vi "FPGA Main Simple Torque.vi"() -> ()   [LabVIEW 2018]
doc: "This VI reads all analogue data channels available at the fastest rate supported by the respective hardware and updates a memory address for when each measurement is available.\n\nAt a rate defined by the fastest module (NI 9237 - default of 12.5kHz) this memory is read, combined with the measurements from the 9237 module and written to the FIFO for communication to the RT machine.\n\nThe NI 9237 modeul therefore defines the nominal sampling rate of the system (with slower channels over-sampled).\n\nA time channel (in uSec) is provided with 0 referenced from the first acquisition of the NI 9237 module"
uses:
  <vilib>/LabVIEW Targets/FPGA/cRIO/shared/nicrio_ModuleControls/nicrio_cRIO-9237_DataRatesRing.ctl
  <vilib>/Platform/TimedLoop/XDataNode/timing_clust.ctl
  <vilib>/Platform/TimedLoop/XDataNode/nitl_modes.ctl
  <vilib>/Platform/TimedLoop/XDataNode/wakeup.ctl
  <vilib>/rvi/Emulation/niFpgaGetClockAttributes.vi
  <vilib>/rvi/Emulation/niFpgaSctlEmulationGetInTimedLoop.vi
  <vilib>/rvi/Emulation/niFpgaEmulationReportErrorSimple.vi
  <vilib>/rvi/Emulation/niFpgaProcessEmulError.vi
  <vilib>/rvi/eio/common/nirviEmuTemplatePropertySet_noerrors.vi
  <vilib>/rvi/eio/common/nirviEmuTemplateMethod_errors.vi
  <vilib>/rvi/interface/RandomDataEmulation/niFpgaRandomDataHandleErrors.vi
  <vilib>/rvi/Memory/Memory_Emulation/nirvimemoryFastEmulation.vi
  <vilib>/rvi/Memory/Memory_Emulation/nirvimemoryEmulation.vi
  <vilib>/rvi/Emulation/niFpgaEmulationIsFPGAContextNoSignature.vi
  <vilib>/rvi/DataTransferAndStorage/Container/Common/niFpgaContainerGetUniqueNameForEmu.vi
  <vilib>/rvi/errors/nirviReportUnexpectedCaseInternalError (U32).vi
  <vilib>/rvi/Emulation/niFpgaCriticalErrorInLSC.vi
  <vilib>/eio/EIOPropertyNode/EIOPropertyNode.xnode
  <vilib>/eio/EIONode/EIONode.xnode
  <vilib>/rvi/DataTransferAndStorage/Container/XNode/niFpgaContainer.xnode
  <vilib>/rvi/interface/RandomDataEmulation/nirviRandomDataFpgaReadWriteTemplate.vi
  <vilib>/platform/TimedLoop/XDataNode/XDataNode.xnode
  <vilib>/eio/EIOMethodNode/EIOMethodNode.xnode
  <vilib>/Platform/TimedLoop/XDataNode/XDNodeRunTimeDep.lvlib
  <vilib>/rvi/eio/common/nirviEmuTemplatePropertyGet_errors.vi
  <vilib>/rvi/eio/common/nirviEmuTemplatePropertyGet_noerrors.vi
  <vilib>/rvi/eio/common/nirviEmuTemplatePropertySet_errors.vi
panel:
  in  "filterTorque":bool
  in  "Data Rate":T1=1 items=["50.000 kS/s (NI 9237)"=1, "25.000 kS/s (NI 9237)"=2, "16.667 kS/s (NI 9237)"=3, "12.500 kS/s (NI 9237)"=4, "10.000 kS/s (NI 9237)"=5, "8.333 kS/s (NI 9237)"=6, "7.143 kS/s (NI 9237)"=7, "6.250 kS/s (NI 9237)"=8, "5.556 kS/s (NI 9237)"=9, "5.000 kS/s (NI 9237)"=10, "4.545 kS/s (NI 9237)"=11, "4.167 kS/s (NI 9237)"=12, "3.846 kS/s (NI 9237)"=13, "3.571 kS/s (NI 9237)"=14, "3.333 kS/s (NI 9237)"=15, "3.125 kS/s (NI 9237)"=16, "2.941 kS/s (NI 9237)"=17, "2.778 kS/s (NI 9237)"=18, "2.632 kS/s (NI 9237)"=19, "2.500 kS/s (NI 9237)"=20, "2.381 kS/s (NI 9237)"=21, "2.273 kS/s (NI 9237)"=22, "2.174 kS/s (NI 9237)"=23, "2.083 kS/s (NI 9237)"=24, "2.000 kS/s (NI 9237)"=25, "1.923 kS/s (NI 9237)"=26, "1.852 kS/s (NI 9237)"=27, "1.786 kS/s (NI 9237)"=28, "1.724 kS/s (NI 9237)"=29, "1.667 kS/s (NI 9237)"=30, "1.613 kS/s (NI 9237)"=31]
  in  "encoders offset":u32 caption="encoder offset @ 1Hz (ticks)"
  out "Total channel count":u32=61
  out "timestamp":u32
  out "FIFO full counter":i32
  in  "Safe Voltage":fxp<+/-,20,5>[](array[numeric])=[0.0, 0.0, 0.0, 0.0]
  in  "Safe Digital":bool[](array[boolean])=[FALSE, FALSE, FALSE, FALSE, FALSE, FALSE, FALSE, FALSE]
  in  "Voltage Out":fxp<+/-,20,5>[](array[numeric])=[0.0, 0.0, 0.0, 0.0]
  in  "Update Outputs":bool
  in  "Mod 8":bool[](array[boolean])=[FALSE, FALSE, FALSE, FALSE, FALSE, FALSE, FALSE, FALSE]
  out "E Stop":bool
  in  "Stop acquire":bool
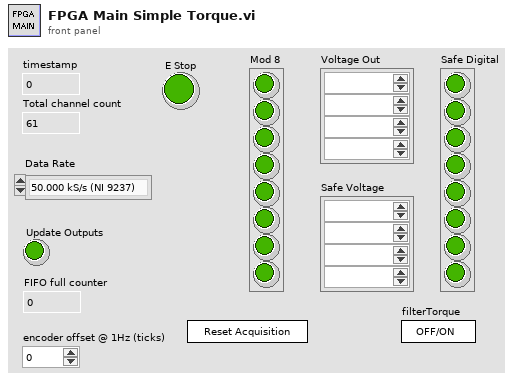
[diagram p1: front panel]
types:
  T1 = typedef "nicrio_cRIO-9237_DataRatesRing.ctl" = u8
  T2 = typedef "XDNodeRunTimeDep.lvlib/timing_clust.ctl" = cluster{"Expected End [f-1]":u64, "Actual End [f-1]":u64, "Finished Late? [f-1]":bool, "Expected End [i-1]":u64, "Actual End [i-1]":u64, "Finished Late? [i-1]":bool, "Expected Start [i]":u64, "Actual Start [i]":u64, "Expected Start [f]":u64, "Actual Start [f]":u64, "Source Name":string, "Structure Name":string, "Period":i64, "Deadline":i64, "Offset":i64, "Start":i64, "Priority":i32, "Timeout":i32, "Mode":T3, "Wakeup Reason":T4, "Error":errorcluster, "Source Type":string, "Secondary Source Type":string, "Global End Time":u64, "Global Start Time":u64, "Frame Duration":u64, "Iteration Duration":u64, "Assigned CPU":i32, "I/O Scan Engine Mode":u32}
  T3 = typedef "XDNodeRunTimeDep.lvlib/nitl_modes.ctl" = enum32{"No Change", "Process missed periods, maintain original phase", "Discard missed periods, maintain original phase", "Process missed periods, ignore original phase", "Discard missed periods, ignore original phase"}
  T4 = typedef "XDNodeRunTimeDep.lvlib/wakeup.ctl" = enum32{"Normal", "Aborted", "Asynchronous wakeup", "Timing source error", "Timed loop error", "Timeout"}
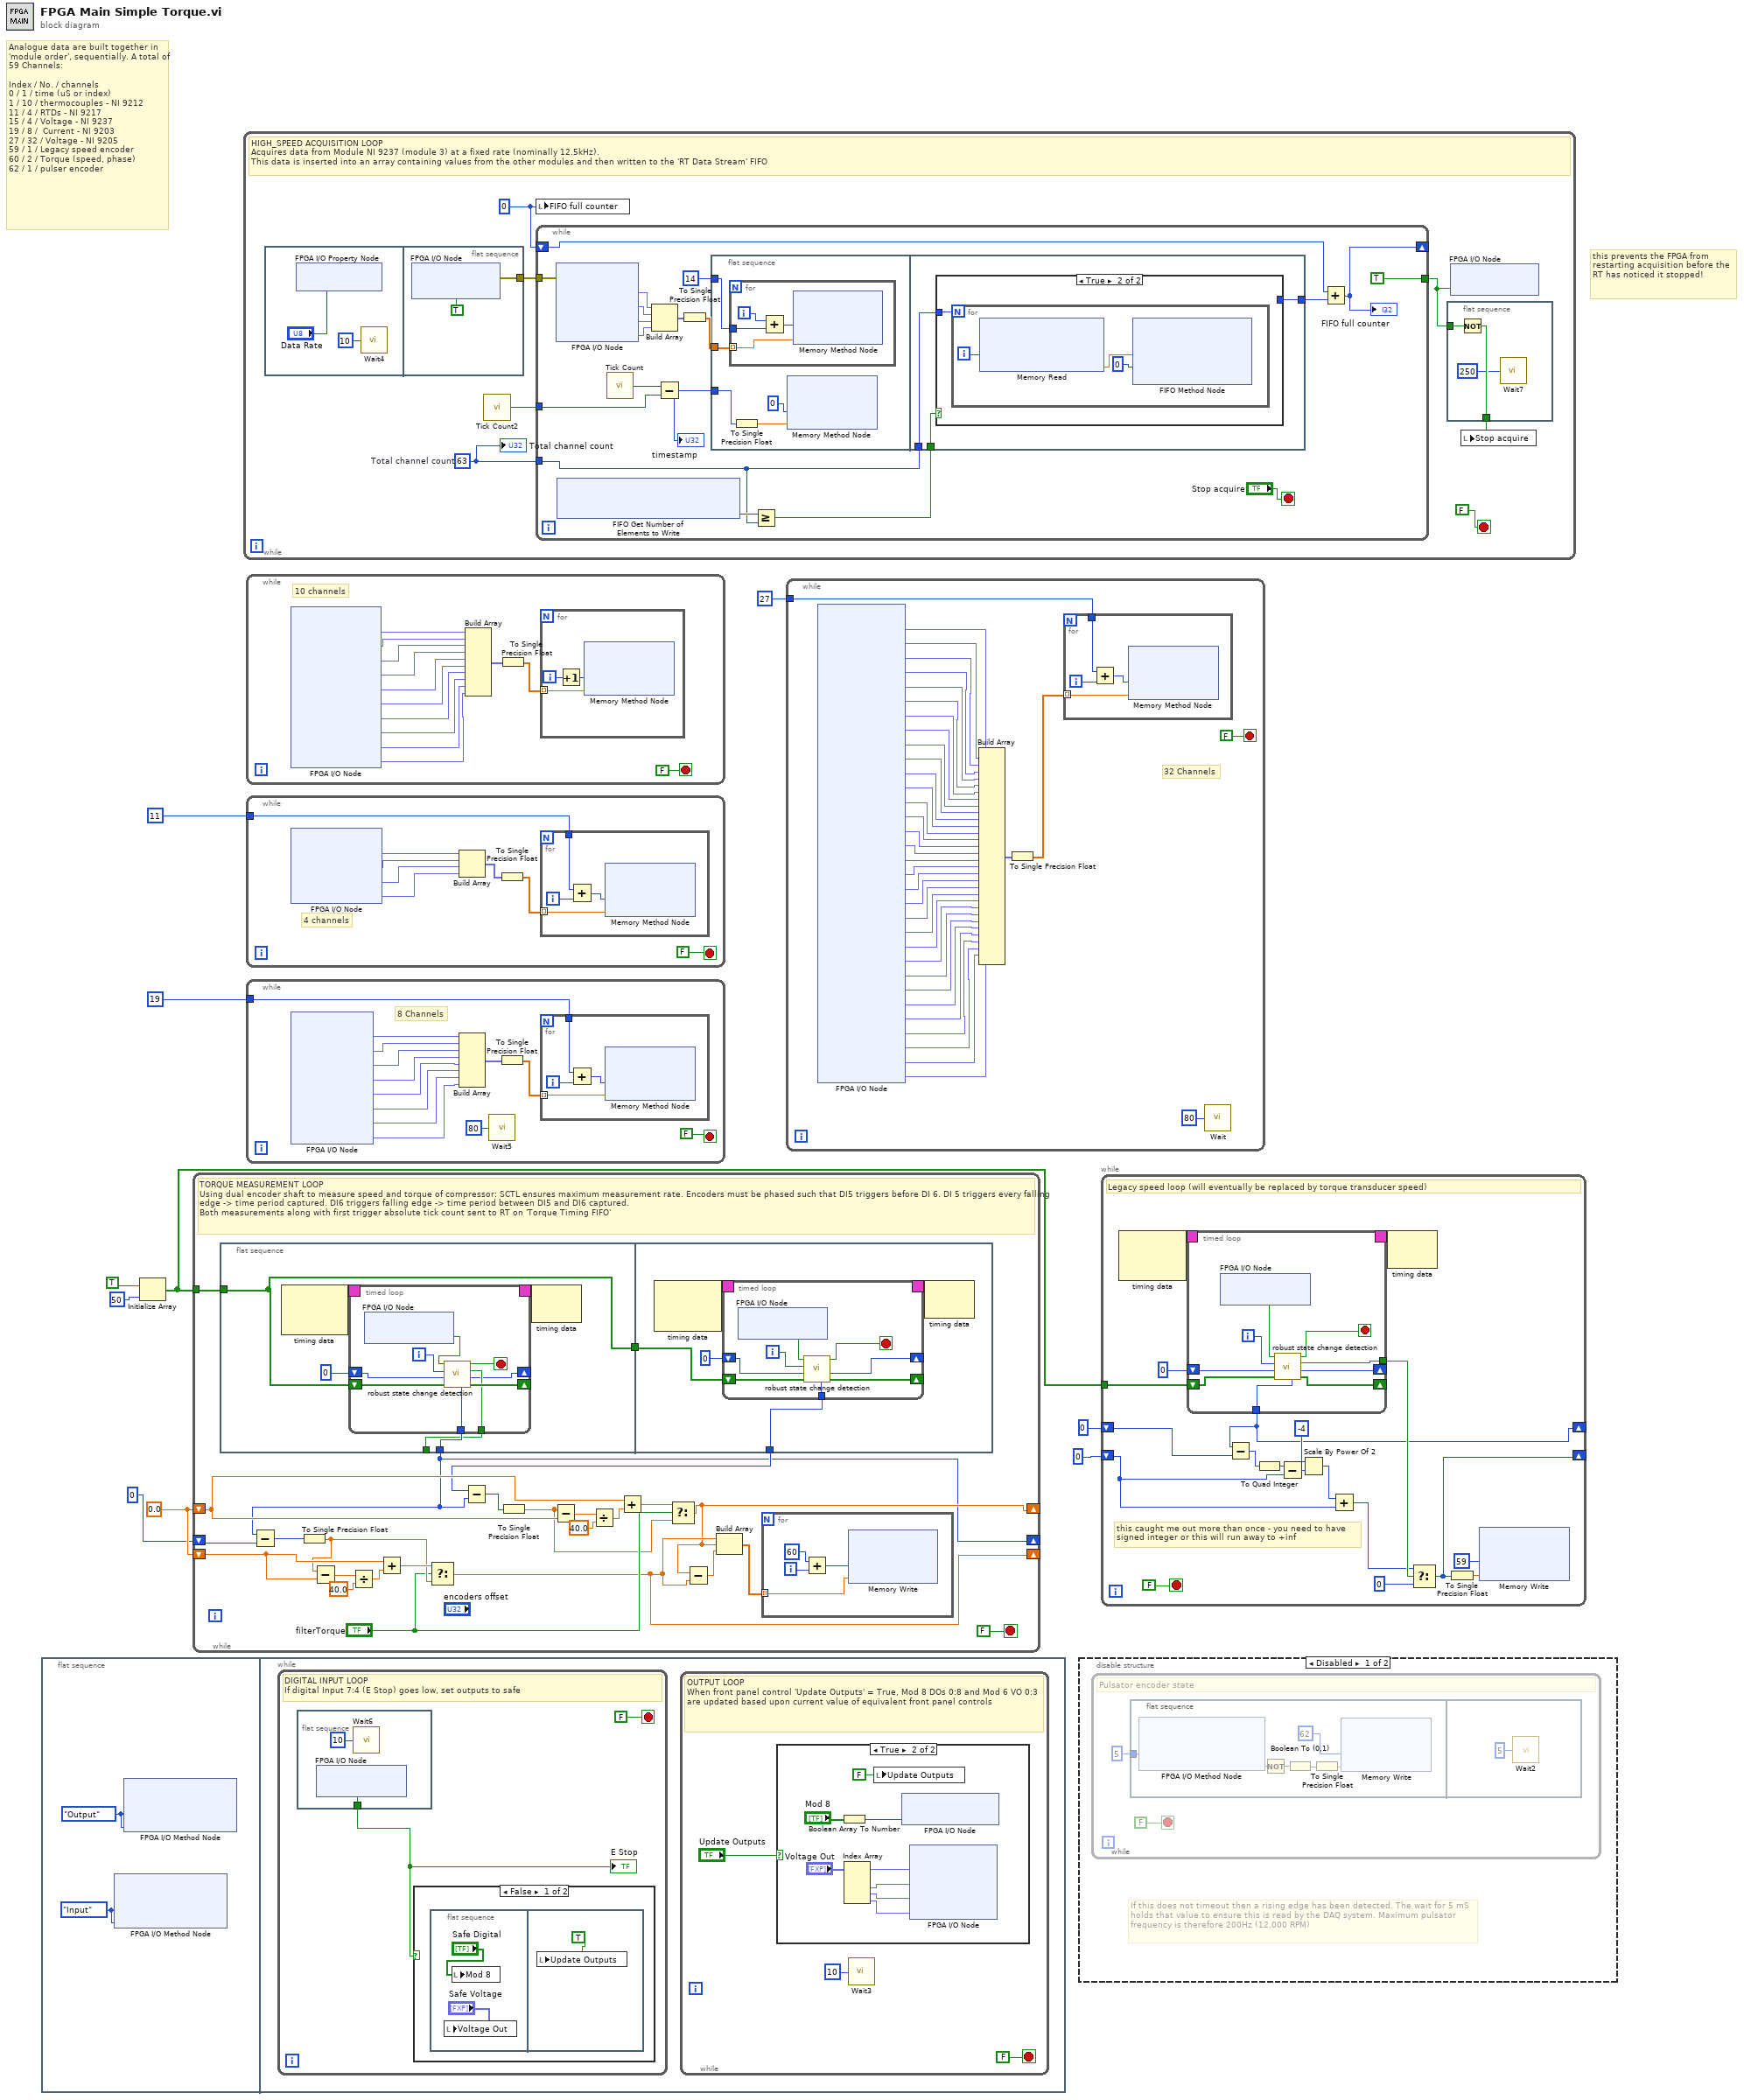
[diagram p0: block diagram]
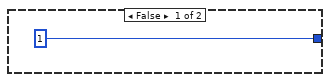
[diagram p5: hidden frame]
diagram:
  w2 = sgl 0.0
  # "this prevents the FPGA from restarting acquisition before the RT has noticed it stopped!"
  # "Analogue data are built together in 'module order', sequentially. A total of 59 Channels:\n\nIndex / No. / channels\n0 / 1 / time (uS or index)\n1 / 10 / thermocouples - NI 9212\n11 / 4 / RTDs - NI 9217\n15 / 4 / Voltage - NI 9237\n19 / 8 /  Current - NI 9203\n27 / 32 / Voltage - NI 9205\n59 / 1 / Legacy speed encoder\n60 / 2 / Torque (speed, phase)\n62 / 1 / pulser encoder"
  n1 = flat-sequence {
    frame #0 {
      w11 = enum8{"No Change", "Input", "Output"}."Output" ("DIO 7:4")
      w12 = enum8{"No Change", "Input", "Output"}."Input" ("DIO 7:4")
      n2 = xnode "FPGA I/O Method Node"("DIO 7:4"=w12, "DIO 3:0"=w12) -> ()  [unwired: 1 in, 1 out]
      n3 = xnode "FPGA I/O Method Node"("DIO 7:4"=w11, "DIO 3:0"=w11) -> ()  [unwired: 1 in, 1 out]
    }
    frame #1 {
      n4 = while {
        stop <- FALSE stop-if-true
        # "DIGITAL INPUT LOOP\nIf digital Input 7:4 (E Stop) goes low, set outputs to safe"
        n5 = flat-sequence {
          tunnel: [w27] -> w24
          frame #0 {
            n6 = xnode "FPGA I/O Node"() -> ("Mod7/DIO4"=w27:bool)  [unwired: 1 in, 1 out]
            n7 = call "Wait6"("Count(uSec)"=u8 10) -> ()  [unwired: 1 out]
          }
        }
        n8 = case shown="False" w24 {
          frame False {
            n9 = flat-sequence {
              frame #0 {
                n10 = local write "Voltage Out"("Safe Voltage") -> ()
                n11 = local write "Mod 8"("Safe Digital") -> ()
              }
              frame #1 {
                n12 = local write "Update Outputs"(TRUE ("Update Outputs")) -> ()
              }
            }
          }
          frame True {
          }
        }
        "E Stop" <- w24
      }
      n13 = while {
        stop <- FALSE stop-if-true
        # "OUTPUT LOOP\nWhen front panel control 'Update Outputs' = True, Mod 8 DOs 0:8 and Mod 6 VO 0:3 are updated based upon current value of equivalent front panel controls"
        n14 = case shown="True" "Update Outputs" {
          frame False {
          }
          frame True {
            n15 = Boolean Array To Number(Boolean array="Mod 8") -> (number=w22:u8)
            n16 = Index Array(array="Voltage Out") -> (element #1=w20:fxp<+/-,20,5>, element #2=w19:fxp<+/-,20,5>, element #3=w18:fxp<+/-,20,5>, element #4=w17:fxp<+/-,20,5>)  [unwired: 4 in]
            n17 = local write "Update Outputs"(FALSE ("Update Outputs")) -> ()
            n18 = xnode "FPGA I/O Node"("Mod8/DIO7:0"=w22) -> ()  [unwired: 1 in, 1 out]
            n19 = xnode "FPGA I/O Node"("Mod6/AO0"=w20, "Mod6/AO1"=w19, "Mod6/AO2"=w18, "Mod6/AO3"=w17) -> ()  [unwired: 4 in, 4 out]
          }
        }
        n20 = call "Wait3"("Count(uSec)"=u16 10 ("Count(Ticks)")) -> ()  [unwired: 1 out]
      }
    }
  }
  n21 = Initialize Array(TRUE, 50 ("edge buffer size")) -> (w4:bool[])
  n22 = while {
    shift-right: [w33] -> _
    shift-left: w2 -> [w43]
    shift-right: [w32] -> _
    shift-left: w2 -> [w53]
    tunnel: w4 -> [w52]
    shift-right: [w31] -> _
    shift-left: u32 0 ("tick") -> [w37]
    stop <- FALSE stop-if-true
    # "TORQUE MEASUREMENT LOOP\nUsing dual encoder shaft to measure speed and torque of compressor: SCTL ensures maximum measurement rate. Encoders must be phased such that DI5 triggers before DI 6. DI 5 triggers every falling edge -> time period captured. DI6 triggers falling edge -> time period between DI5 and DI6 captured.\nBoth measurements along with first trigger absolute tick count sent to RT on 'Torque Timing FIFO'"
    n23 = flat-sequence {
      tunnel: [w63] -> w31
      tunnel: [w62] -> _
      tunnel: w52 -> [w60]
      tunnel: [w60] -> w51
      tunnel: [w83] -> w34
      tunnel: w51 -> [w82]
      frame #0 {
        n24 = node-c288() -> (w65:T2)  [unwired: 2 in]
        n25 = timed-loop {
          timing: w65 -> [_]
          timing-out: [_] -> w64
          tunnel: [w69] -> w63
          tunnel: [w68] -> w62
          shift-right: [w72] -> _
          shift-left: w60 -> [w73]
          shift-right: [w66] -> _
          shift-left: i16 0 ("step") -> [w70]
          i -> [w71]
          stop <- w67 stop-if-true
          n26 = xnode "FPGA I/O Node"() -> ("Mod7/DIO0"=w74:bool)  [unwired: 1 in, 1 out]
          n27 = call "robust state change detection.vi"("history"=w73, "step"=w70, "tick"=w71, "New state"=w74) -> ("history out"=w72:bool[], "step out"=w66:i16, "edge detected"=w68:bool, "Stop?"=w67:bool, "tick"=w69:u32)  [unwired: 3 in]
        }
        n28 = node-c288(w64) -> ()  [unwired: 1 out]
      }
      frame #1 {
        n29 = node-c288() -> (w81:T2)  [unwired: 2 in]
        n30 = timed-loop {
          timing: w81 -> [_]
          timing-out: [_] -> w80
          shift-right: [w89] -> _
          shift-left: w82 -> [w90]
          tunnel: [w87] -> w83
          shift-right: [w84] -> _
          shift-left: i16 0 ("step") -> [w85]
          i -> [w86]
          stop <- w88 stop-if-true
          n31 = xnode "FPGA I/O Node"() -> ("Mod7/DIO1"=w91:bool)  [unwired: 1 in, 1 out]
          n32 = call "robust state change detection.vi"("history"=w90, "step"=w85, "tick"=w86, "New state"=w91) -> ("history out"=w89:bool[], "step out"=w84:i16, "Stop?"=w88:bool, "tick"=w87:u32)  [unwired: 3 in, 1 out]
        }
        n33 = node-c288(w80) -> ()  [unwired: 1 out]
      }
    }
    n34 = Subtract(x=w31, y=w37) -> (x-y=w36:u32)
    n35 = To Single Precision Float(number=w36) -> (single precision float=w41:sgl)
    n36 = Subtract(x=w41, y=w43) -> (x-y=w44:sgl)
    n37 = Divide(x=w44, y=sgl 40.0) -> (x/y=w45:sgl)
    n38 = Add(x=w43, y=w45) -> (x+y=w46:sgl)
    n39 = Select(t=w46, s="filterTorque", f=w41) -> (s? t:f=w33:sgl)
    n40 = Subtract(x=w34, y=w31) -> (x-y=w35:u32)
    n41 = To Single Precision Float(number=w35) -> (single precision float=w39:sgl)
    n42 = Subtract(x=w39, y=w53) -> (x-y=w50:sgl)
    n43 = Divide(x=w50, y=sgl 40.0) -> (x/y=w48:sgl)
    n44 = Add(x=w53, y=w48) -> (x+y=w47:sgl)
    n45 = Select(t=w47, s="filterTorque", f=w39) -> (s? t:f=w32:sgl)
    n46 = Subtract(x=w32, y=w33) -> (x-y=w38:sgl)
    n47 = Build Array(w33, w32, w38) -> (w54:sgl[])
    n48 = for {
      tunnel: w54 -> [w56] mode=indexing
      i -> [w57]
      n49 = Add(x=u32 60 ("Address"), y=w57) -> (x+y=w58:u32)
      n50 = xnode ("Memory Write")("Address"=w58, "Data"=w56) -> ()  [unwired: 1 in, 1 out]
    }
  }
  n51 = while {
    stop <- FALSE stop-if-true
    w97 = 0 ("FIFO full counter")
    w100 = u32 63  # Total channel count
    # "HIGH_SPEED ACQUISITION LOOP\nAcquires data from Module NI 9237 (module 3) at a fixed rate (nominally 12.5kHz).\nThis data is inserted into an array containing values from the other modules and then written to the 'RT Data Stream' FIFO"
    n52 = flat-sequence {
      tunnel: [w109] -> w101
      frame #0 {
        n53 = xnode "FPGA I/O Property Node"("Data Rate"="Data Rate") -> ()  [unwired: 1 in, 1 out]
        n54 = call "Wait4"("Count(mSec)"=u16 10) -> ()  [unwired: 1 out]
      }
      frame #1 {
        n55 = xnode "FPGA I/O Node"("Mod3/Start"=TRUE) -> ("error out"=w109:errorcluster)  [unwired: 2 in, 1 out]
      }
    }
    n56 = call "Tick Count2"() -> ("Tick Count(uSec)"=w102:u32)
    n57 = local write "FIFO full counter"(w97) -> ()
    n58 = while {
      tunnel: [TRUE ("I/O Item")] -> w99
      tunnel: w101 -> [w127]
      tunnel: w100 -> [w112]
      shift-right: [w120] -> _
      shift-left: w97 -> [w118]
      tunnel: w102 -> [w121]
      stop <- "Stop acquire" stop-if-true
      n59 = xnode "FPGA I/O Node"("error in"=w127) -> ("Mod3/AI0"=w126:fxp<+/-,24,-4>, "Mod3/AI1"=w125:fxp<+/-,24,-4>, "Mod3/AI2"=w124:fxp<+/-,24,-4>, "Mod3/AI3"=w123:fxp<+/-,24,-4>)  [unwired: 4 in, 5 out]
      n60 = xnode ("FIFO Get Number of Elements to Write")() -> ("Number of Elements to Write"=w114:u32)  [unwired: 1 in, 1 out]
      n61 = call "Tick Count"() -> ("Tick Count(uSec)"=w117:u32)
      n62 = Build Array(w126, w125, w124, w123) -> (w122:fxp<+/-,24,-4>[])
      n63 = Subtract(x=w117, y=w121) -> (x-y=w110:u32)
      "timestamp" <- w110
      n64 = To Single Precision Float(number=w122) -> (single precision float=w116:sgl[])
      n65 = flat-sequence {
        tunnel: w116 -> [w133]
        tunnel: 14 ("index") -> [w132]
        tunnel: w110 -> [w130]
        tunnel: w112 -> [w140]
        tunnel: [w139] -> w111
        tunnel: w113 -> [w138]
        frame #0 {
          n66 = for {
            tunnel: w133 -> [w137] mode=indexing
            tunnel: w132 -> [w136]
            i -> [w134]
            n67 = Add(x=w134, y=w136) -> (x+y=w135:i32)
            n68 = xnode ("Memory Method Node")("Address"=w135, "Data"=w137) -> ()  [unwired: 1 in, 1 out]
          }
          n69 = To Single Precision Float(number=w130) -> (single precision float=w131:sgl)
          n70 = xnode ("Memory Method Node")("Address"=u32 0, "Data"=w131) -> ()  [unwired: 1 in, 1 out]
        }
        frame #1 {
          n71 = case shown="True" w138 {
            tunnel: [1 _] -> w139
            tunnel: w140 -> [_ w142]
            frame False {
            }
            frame True {
              n72 = for {
                N: w142 -> [_]
                i -> [w143]
                n73 = xnode ("Memory Read")("Address"=w143) -> ("Data"=w144:sgl)  [unwired: 1 in, 1 out]
                n74 = xnode ("FIFO Method Node")("Element"=w144, "Timeout"=0) -> ()  [unwired: 1 in, 2 out]
              }
            }
          }
        }
      }
      n75 = Greater Or Equal?(x=w114, y=w112) -> (x >= y?=w113:bool)
      n76 = Add(x=w118, y=w111) -> (x+y=w120:i32)
      "FIFO full counter" <- w120
    }
    n77 = flat-sequence {
      tunnel: w99 -> [w105]
      tunnel: [w104] -> w96
      frame #0 {
        n78 = Not(x=w105) -> (.not. x?=w104:bool)
        n79 = call "Wait7"("Count(mSec)"=u8 250) -> ()  [unwired: 1 out]
      }
    }
    n80 = xnode "FPGA I/O Node"("Mod3/Stop"=w99) -> ()  [unwired: 1 in, 1 out]
    n81 = local write "Stop acquire"(w96) -> ()
    "Total channel count" <- w100
  }
  n82 = while {
    stop <- FALSE stop-if-true
    # "10 channels"
    n83 = xnode "FPGA I/O Node"() -> ("Mod1/TC0"=w158:fxp<+/-,24,-2>, "Mod1/TC1"=w157:fxp<+/-,24,-2>, "Mod1/TC2"=w156:fxp<+/-,24,-2>, "Mod1/TC3"=w155:fxp<+/-,24,-2>, "Mod1/TC4"=w154:fxp<+/-,24,-2>, "Mod1/TC5"=w153:fxp<+/-,24,-2>, "Mod1/TC6"=w152:fxp<+/-,24,-2>, "Mod1/TC7"=w151:fxp<+/-,24,-2>, "Mod1/CJC0"=w148:fxp<+/-,24,-2>, "Mod1/CJC1"=w147:fxp<+/-,24,-2>)  [unwired: 10 in, 10 out]
    n84 = Build Array(w158, w157, w156, w155, w154, w153, w152, w151, w148, w147) -> (w150:fxp<+/-,24,-2>[])
    n85 = To Single Precision Float(number=w150) -> (single precision float=w149:sgl[])
    n86 = for {
      tunnel: w149 -> [w161] mode=indexing
      i -> [w160]
      n87 = Increment(x=w160) -> (x+1=w159:i32)
      n88 = xnode ("Memory Method Node")("Address"=w159, "Data"=w161) -> ()  [unwired: 1 in, 1 out]
    }
  }
  n89 = while {
    tunnel: 11 ("Numeric") -> [w163]
    stop <- FALSE stop-if-true
    # "4 channels"
    n90 = xnode "FPGA I/O Node"() -> ("Mod2/RTD0"=w169:fxp<+/-,24,10>, "Mod2/RTD1"=w168:fxp<+/-,24,10>, "Mod2/RTD2"=w167:fxp<+/-,24,10>, "Mod2/RTD3"=w164:fxp<+/-,24,10>)  [unwired: 4 in, 4 out]
    n91 = Build Array(w169, w168, w167, w164) -> (w166:fxp<+/-,24,10>[])
    n92 = To Single Precision Float(number=w166) -> (single precision float=w165:sgl[])
    n93 = for {
      tunnel: w165 -> [w173] mode=indexing
      tunnel: w163 -> [w170]
      i -> [w172]
      n94 = Add(x=w170, y=w172) -> (x+y=w171:i32)
      n95 = xnode ("Memory Method Node")("Address"=w171, "Data"=w173) -> ()  [unwired: 1 in, 1 out]
    }
  }
  n96 = while {
    tunnel: 19 ("Numeric") -> [w180]
    stop <- FALSE stop-if-true
    # "8 Channels"
    n97 = xnode "FPGA I/O Node"() -> ("Mod4/AI0"=w186:fxp<+/-,21,-4>, "Mod4/AI1"=w185:fxp<+/-,21,-4>, "Mod4/AI2"=w184:fxp<+/-,21,-4>, "Mod4/AI3"=w181:fxp<+/-,21,-4>, "Mod4/AI4"=w179:fxp<+/-,21,-4>, "Mod4/AI5"=w178:fxp<+/-,21,-4>, "Mod4/AI6"=w177:fxp<+/-,21,-4>, "Mod4/AI7"=w176:fxp<+/-,21,-4>)  [unwired: 8 in, 8 out]
    n98 = Build Array(w186, w185, w184, w181, w179, w178, w177, w176) -> (w183:fxp<+/-,21,-4>[])
    n99 = call "Wait5"("Count(uSec)"=u8 80) -> ()  [unwired: 1 out]
    n100 = To Single Precision Float(number=w183) -> (single precision float=w182:sgl[])
    n101 = for {
      tunnel: w182 -> [w190] mode=indexing
      tunnel: w180 -> [w187]
      i -> [w189]
      n102 = Add(x=w187, y=w189) -> (x+y=w188:i32)
      n103 = xnode ("Memory Method Node")("Address"=w188, "Data"=w190) -> ()  [unwired: 1 in, 1 out]
    }
  }
  n104 = while {
    tunnel: 27 ("Numeric") -> [w226]
    stop <- FALSE stop-if-true
    # "32 Channels"
    n105 = xnode "FPGA I/O Node"() -> ("Mod5/AI0"=w194:fxp<+/-,26,5>, "Mod5/AI1"=w195:fxp<+/-,26,5>, "Mod5/AI2"=w196:fxp<+/-,26,5>, "Mod5/AI3"=w197:fxp<+/-,26,5>, "Mod5/AI4"=w198:fxp<+/-,26,5>, "Mod5/AI5"=w199:fxp<+/-,26,5>, "Mod5/AI6"=w200:fxp<+/-,26,5>, "Mod5/AI7"=w201:fxp<+/-,26,5>, "Mod5/AI8"=w225:fxp<+/-,26,5>, "Mod5/AI9"=w224:fxp<+/-,26,5>, "Mod5/AI10"=w223:fxp<+/-,26,5>, "Mod5/AI11"=w222:fxp<+/-,26,5>, "Mod5/AI12"=w221:fxp<+/-,26,5>, "Mod5/AI13"=w220:fxp<+/-,26,5>, "Mod5/AI14"=w219:fxp<+/-,26,5>, "Mod5/AI15"=w218:fxp<+/-,26,5>, "Mod5/AI16"=w217:fxp<+/-,26,5>, "Mod5/AI17"=w216:fxp<+/-,26,5>, "Mod5/AI18"=w215:fxp<+/-,26,5>, "Mod5/AI19"=w214:fxp<+/-,26,5>, "Mod5/AI20"=w213:fxp<+/-,26,5>, "Mod5/AI21"=w212:fxp<+/-,26,5>, "Mod5/AI22"=w211:fxp<+/-,26,5>, "Mod5/AI23"=w210:fxp<+/-,26,5>, "Mod5/AI24"=w209:fxp<+/-,26,5>, "Mod5/AI25"=w208:fxp<+/-,26,5>, "Mod5/AI26"=w207:fxp<+/-,26,5>, "Mod5/AI27"=w206:fxp<+/-,26,5>, "Mod5/AI28"=w205:fxp<+/-,26,5>, "Mod5/AI29"=w204:fxp<+/-,26,5>, "Mod5/AI30"=w203:fxp<+/-,26,5>, "Mod5/AI31"=w202:fxp<+/-,26,5>)  [unwired: 32 in, 32 out]
    n106 = Build Array(w194, w195, w196, w197, w198, w199, w200, w201, w225, w224, w223, w222, w221, w220, w219, w218, w217, w216, w215, w214, w213, w212, w211, w210, w209, w208, w207, w206, w205, w204, w203, w202) -> (w227:fxp<+/-,26,5>[])
    n107 = To Single Precision Float(number=w227) -> (single precision float=w193:sgl[])
    n108 = for {
      tunnel: w193 -> [w231] mode=indexing
      tunnel: w226 -> [w228]
      i -> [w230]
      n109 = Add(x=w228, y=w230) -> (x+y=w229:i32)
      n110 = xnode ("Memory Method Node")("Address"=w229, "Data"=w231) -> ()  [unwired: 1 in, 1 out]
    }
    n111 = call "Wait"("Count(uSec)"=u8 80) -> ()  [unwired: 1 out]
  }
  n112 = disable-structure shown="Disabled" {
    frame Disabled {
      # "If this does not timeout then a rising edge has been detected. The wait for 5 mS holds that value to ensure this is read by the DAQ system. Maximum pulsator frequency is therefore 200Hz (12,000 RPM)"
      n113 = while {
        stop <- FALSE stop-if-true
        # "Pulsator encoder state"
        n114 = flat-sequence {
          tunnel: 5 ("Timeout") -> [w236]
          frame #0 {
            n115 = xnode "FPGA I/O Method Node"("Timeout"=w236) -> ("Timed Out"=w235:bool)  [unwired: 1 in, 1 out]
            n116 = Not(x=w235) -> (.not. x?=w234:bool)
            n117 = Boolean To (0,1)(Boolean=w234) -> (0, 1=w239:i16)
            n118 = To Single Precision Float(number=w239) -> (single precision float=w238:sgl)
            n119 = xnode ("Memory Write")("Address"=u32 62, "Data"=w238) -> ()  [unwired: 1 in, 1 out]
          }
          frame #1 {
            n120 = call "Wait2"("Count(mSec)"=u16 5 ("Count(uSec)")) -> ()  [unwired: 1 out]
          }
        }
      }
    }
    frame Enabled {
    }
  }
  n121 = while {
    shift-right: [w246] -> _
    shift-left: i64 0 -> [w253]
    tunnel: w4 -> [w247]
    shift-right: [w242] -> _
    shift-left: u32 0 ("tick") -> [w241]
    stop <- FALSE stop-if-true
    # "this caught me out more than once - you need to have signed integer or this will run away to +inf"
    # "Legacy speed loop (will eventually be replaced by torque transducer speed)"
    n122 = node-c288() -> (w259:T2)  [unwired: 2 in]
    n123 = timed-loop {
      timing: w259 -> [_]
      timing-out: [_] -> w258
      shift-right: [w265] -> _
      shift-left: i16 0 ("step") -> [w266]
      tunnel: [w263] -> w248
      tunnel: [w262] -> w242
      shift-right: [w260] -> _
      shift-left: w247 -> [w261]
      i -> [w267]
      stop <- w264 stop-if-true
      n124 = xnode "FPGA I/O Node"() -> ("Mod7/DIO3"=w268:bool)  [unwired: 1 in, 1 out]
      n125 = call "robust state change detection.vi"("history"=w261, "step"=w266, "tick"=w267, "New state"=w268) -> ("history out"=w260:bool[], "step out"=w265:i16, "edge detected"=w263:bool, "Stop?"=w264:bool, "tick"=w262:u32)  [unwired: 3 in]
    }
    n126 = Subtract(x=w242, y=w241) -> (x-y=w243:u32)
    n127 = To Quad Integer(1:w243) -> (0:w250:i64)
    n128 = Subtract(x=w250, y=w253) -> (x-y=w254:i64)
    n129 = Scale By Power Of 2(n=i16 -4, x=w254) -> (x*2^n=w256:i64)
    n130 = Add(x=w256, y=w253) -> (x+y=w244:i64)
    n131 = node-c288(w258) -> ()  [unwired: 1 out]
    n132 = Select(t=w244, s=w248, f=u32 0 ("t")) -> (s? t:f=w246:i64)
    n133 = To Single Precision Float(number=w246) -> (single precision float=w252:sgl)
    n134 = xnode ("Memory Write")("Address"=u32 59, "Data"=w252) -> ()  [unwired: 1 in, 1 out]
  }
